vi "Valid_Bookout.vi"(11 "Bookout List":T1[](array[typedef]) {"End Time" format="%<%d/%m/%Y\n%I:%M:%S %p>T"; "Start Time" format="%<%d/%m/%Y\n%I:%M:%S %p>T"}) -> (3 "Invalid?":bool)   [LabVIEW 2020]
uses:
  Controls/Breakdown_List.ctl
  Controls/Loss_type.ctl
  <userlib>/_OpenG.lib/array/array.llb/Search 1D Array (Boolean)__ogtk.vi
  <userlib>/_OpenG.lib/array/array.llb/Index 1D Array Elements (I32)__ogtk.vi
  <userlib>/_OpenG.lib/array/array.llb/Index 1D Array Elements (String)__ogtk.vi
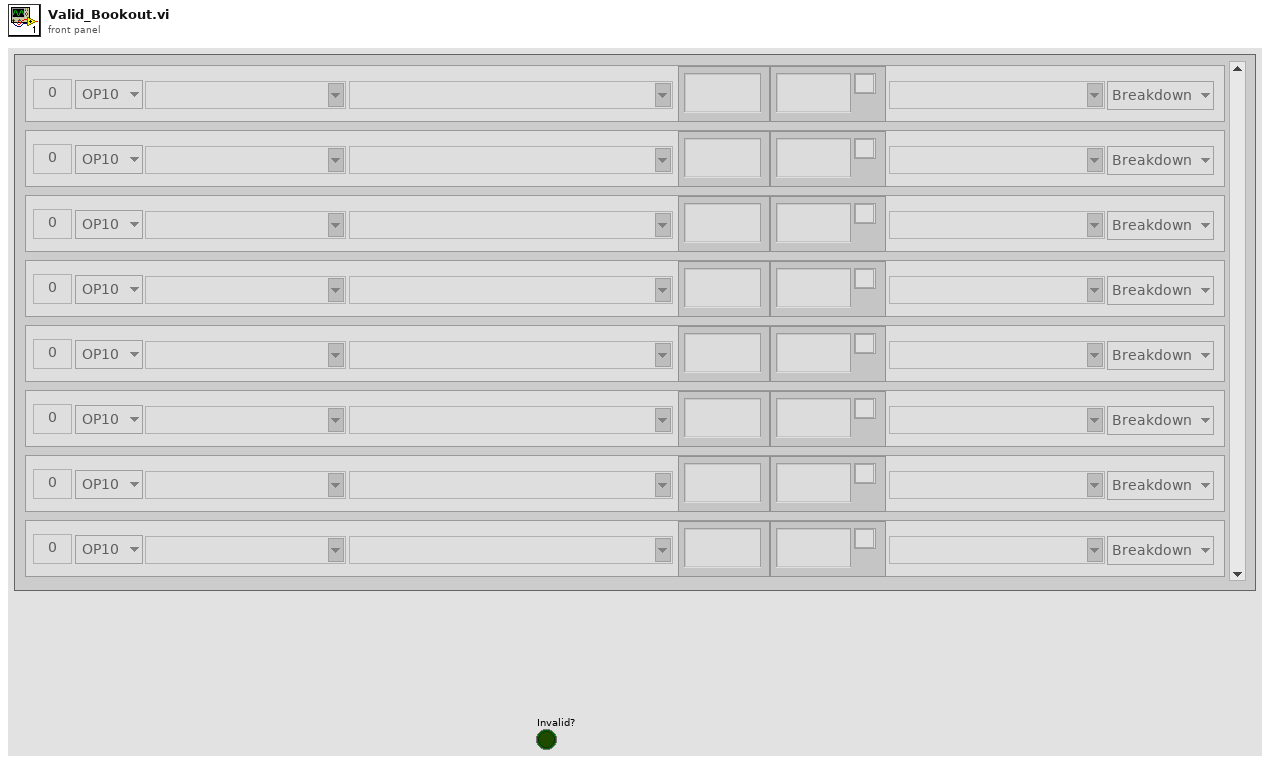
[diagram p1: front panel]
types:
  T1 = typedef "Breakdown_List.ctl" = cluster{"S.No":i32, "Reason Code":string, "Start Time":timestamp, "End Time":timestamp, "Operator":string, "Type":T2, "Machine":enum16{"OP10", "OP20", "OP30", "OP40", "OP50", "OP60", "OP70", "OP80", "LINE"}, "Reason":string}
  T2 = typedef "Loss_type.ctl" = enum16{"Breakdown", "Bookout"}
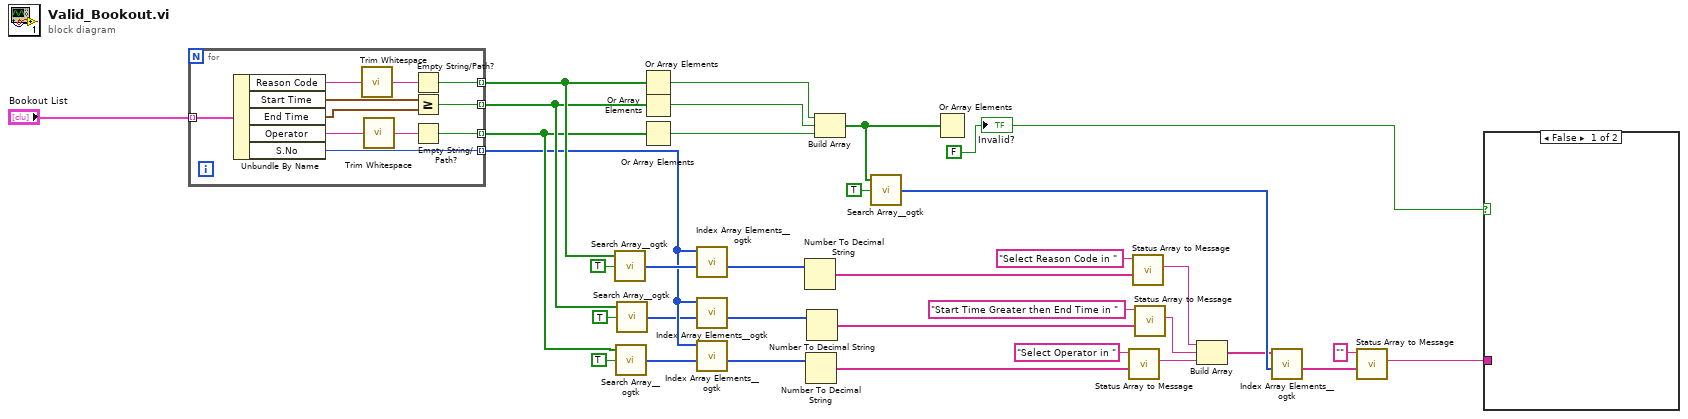
[diagram p0: block diagram]
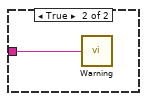
[diagram p2: hidden frame]
diagram:
  w1 = FALSE ("Element Data")
  n1 = for {
    tunnel: "Bookout List" -> [w45] mode=indexing
    tunnel: [w38] -> w30 mode=indexing
    tunnel: [w37] -> w23 mode=indexing
    tunnel: [w36] -> w21 mode=indexing
    tunnel: [w35] -> w11 mode=indexing
    n2 = Unbundle By Name(w45) -> ("Reason Code"=w44:string, "Start Time"=w42:timestamp, "End Time"=w41:timestamp, "Operator"=w39:string, "S.No"=w35:i32)
    n3 = call <vilib>:"Trim Whitespace.vi"("string"=w44) -> ("trimmed string"=w43:string)  [unwired: 1 in]
    n4 = call <vilib>:"Trim Whitespace.vi"("string"=w39) -> ("trimmed string"=w40:string)  [unwired: 1 in]
    n5 = Empty String/Path?(string/path=w43) -> (empty?=w38:bool)
    n6 = Greater Or Equal?(x=w42, y=w41) -> (x >= y?=w37:bool)
    n7 = Empty String/Path?(string/path=w40) -> (empty?=w36:bool)
  }
  n8 = call-poly <userlib>:"Search Array__ogtk.vi"("Array"=w30, "Element Data"=TRUE) -> ("Indices of Elements"=w13:i32[])  [unwired: 7 in]
  n9 = call-poly <userlib>:"Search Array__ogtk.vi"("Array"=w21, "Element Data"=TRUE) -> ("Indices of Elements"=w9:i32[])  [unwired: 7 in]
  n10 = call-poly <userlib>:"Search Array__ogtk.vi"("Array"=w23, "Element Data"=TRUE) -> ("Indices of Elements"=w8:i32[])  [unwired: 7 in]
  n11 = Or Array Elements(Boolean array=w30) -> (logical OR=w33:bool)
  n12 = Or Array Elements(Boolean array=w23) -> (logical OR=w32:bool)
  n13 = Or Array Elements(Boolean array=w21) -> (logical OR=w31:bool)
  n14 = call-poly <userlib>:"Index Array Elements__ogtk.vi"("indices"=w13, "array"=w11) -> ("elements"=w12:i32[])  [unwired: 9 in]
  n15 = call-poly <userlib>:"Index Array Elements__ogtk.vi"("indices"=w8, "array"=w11) -> ("elements"=w10:i32[])  [unwired: 9 in]
  n16 = call-poly <userlib>:"Index Array Elements__ogtk.vi"("indices"=w9, "array"=w11) -> ("elements"=w7:i32[])  [unwired: 9 in]
  n17 = Number To Decimal String(number=w12) -> (decimal integer string=w27:string[])  [unwired: 1 in]
  n18 = Number To Decimal String(number=w7) -> (decimal integer string=w19:string[])  [unwired: 1 in]
  n19 = Number To Decimal String(number=w10) -> (decimal integer string=w26:string[])  [unwired: 1 in]
  n20 = Build Array(w33, w32, w31) -> (w5:bool[])
  n21 = call-poly <userlib>:"Search Array__ogtk.vi"("Array"=w5, "Element Data"=TRUE) -> ("Indices of Elements"=w4:i32[])  [unwired: 7 in]
  n22 = Or Array Elements(Boolean array=w5) -> ()  [unwired: 1 out]
  n23 = call <userlib>:"Status Array to Message.vi"("Status Array"=w19, "Message"="Select Operator in ") -> ("Message"=w16:string)  [unwired: 9 in]
  n24 = call <userlib>:"Status Array to Message.vi"("Status Array"=w27, "Message"="Select Reason Code in ") -> ("Message"=w18:string)  [unwired: 9 in]
  n25 = call <userlib>:"Status Array to Message.vi"("Status Array"=w26, "Message"="Start Time Greater then End Time in ") -> ("Message"=w17:string)  [unwired: 9 in]
  n26 = Build Array(w18, w17, w16) -> (w3:string[])
  n27 = call-poly <userlib>:"Index Array Elements__ogtk.vi"("indices"=w4, "array"=w3) -> ("elements"=w2:string[])  [unwired: 9 in]
  n28 = call <userlib>:"Status Array to Message.vi"("Status Array"=w2, "Message"="") -> ("Message"=w14:string)  [unwired: 9 in]
  n29 = case shown="False" w1 {
    tunnel: w14 -> [_ w46]
    frame False {
    }
    frame True {
      n30 = call <userlib>:"Warning .vi"("Warning in"=w46) -> ()  [unwired: 15 in]
    }
  }
  "Invalid?" <- w1
